vi "Práctica10_ProyectoFinal.vi"() -> ()   [LabVIEW 2021]
panel:
  out "Slide 3":u8(slide) scale=0.0..100.0
  out "Boolean 2":bool
  out "Slide 6":u8(slide) scale=0.0..100.0
  out "Boolean":bool
  out "Acorte 3":dbl(slide) scale=0.0..10.0
  out "Acorte 2":dbl(slide) scale=0.0..10.0
  out "Acorte":dbl(slide) scale=0.0..10.0
  out "Slide 5":u8(slide)
  out "Slide 5":u8(slide)
  out "Slide 5":u8(slide)
  in  "Tipo de papel":string(combo)
  out "Horno":dbl(knob) scale=0.0..100.0
  out "Lignina":dbl(slide) scale=0.0..500.0
  out "Lignina":bool
  out "Slide 5":u8(slide)
  out "Corte":bool
  out "Aplanado":bool
  out "Peroxido":dbl(slide) scale=0.0..500.0
  out "Slide 4":u8(slide)
  out "Slide 5":u8(slide)
  out "Blanquear":bool
  out "Limpieza":bool
  out "Slide 2":u8(slide) scale=0.0..4.0
  out "Distribución":bool
  out "Slide":u8(slide) scale=0.0..10.0 scale format="%_1g"
  out "Almacén":dbl(slide) scale=0.0..100.0
  out "Inicio":bool
  in  "Color Box":u32(colorbox)
  # "Tipo de papel"
  # "Almacén"
  # "Eliminado de lignina"
  # "Triturado"
  # "Aplanado"
  # "Blanqueado"
  # "Cortado"
  # "Distribuido"
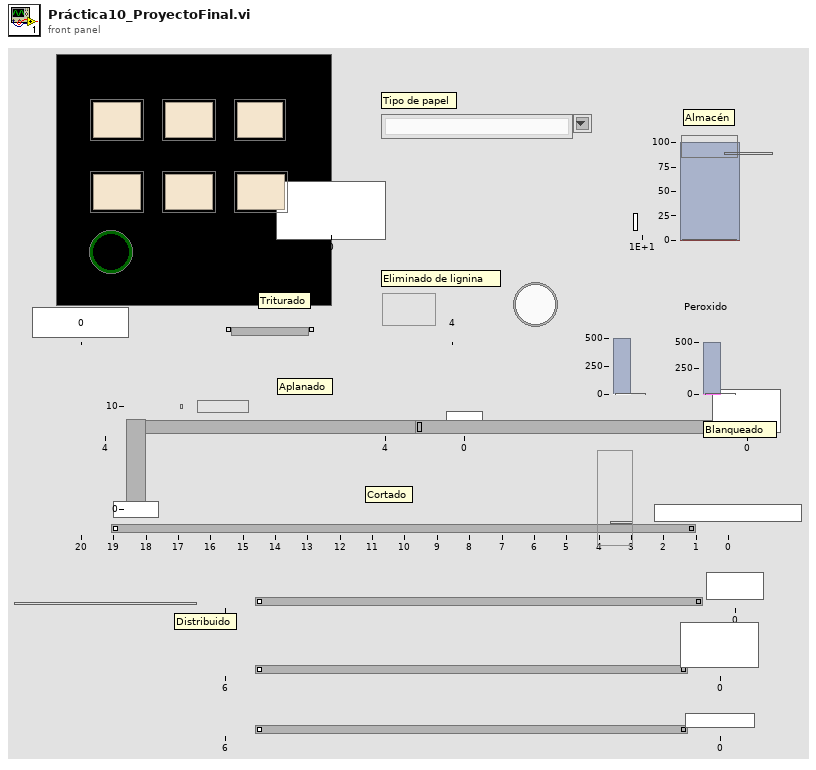
[diagram p1: front panel]
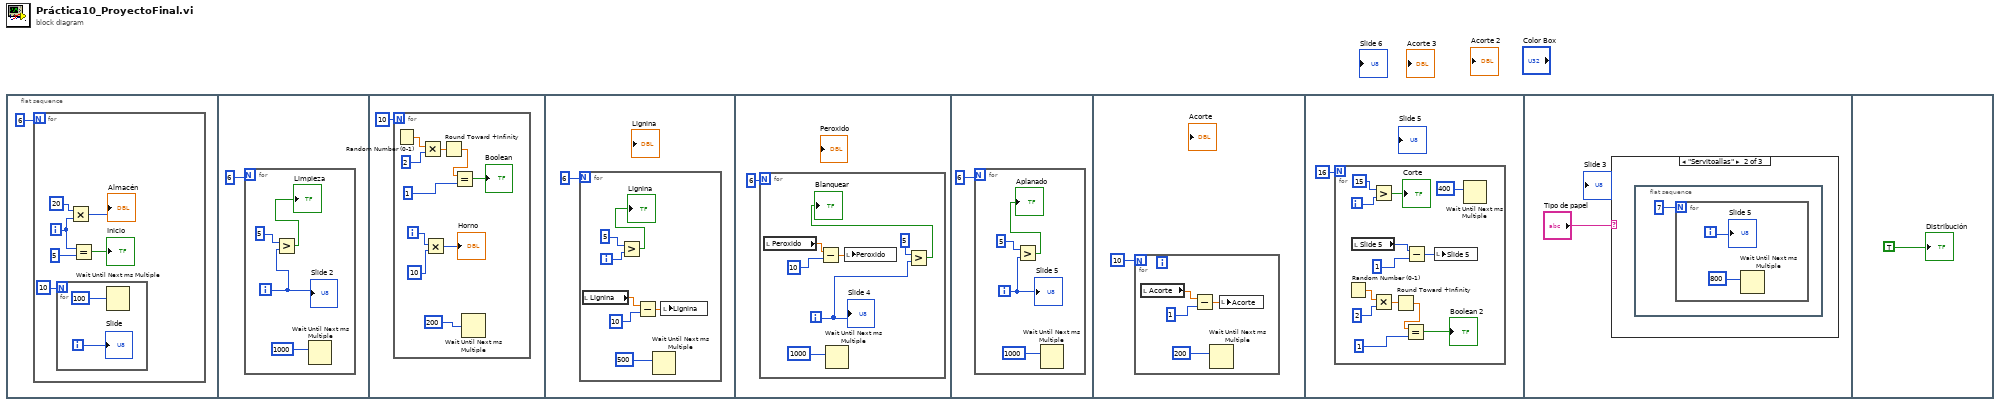
[diagram p0: block diagram]
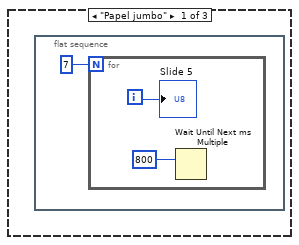
[diagram p2: hidden frame]
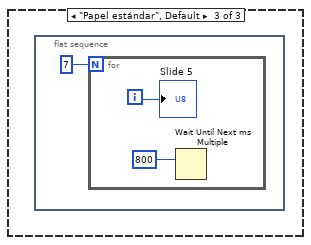
[diagram p3: hidden frame]
diagram:
  n1 = flat-sequence {
    frame #0 {
      n2 = for {
        N: 6 -> [_]
        i -> [w4]
        n3 = for {
          N: 10 -> [_]
          i -> [w8]
          n4 = Wait Until Next ms Multiple(millisecond multiple=100) -> ()  [unwired: 1 out]
          "Slide" <- w8
        }
        n5 = Multiply(x=20, y=w4) -> (x*y=→"Almacén":i32)
        n6 = Equal?(x=w4, y=5) -> (x = y?=→"Inicio":bool)
      }
    }
    frame #1 {
      n7 = for {
        N: 6 -> [_]
        i -> [w12]
        n8 = Greater?(x=5, y=w12) -> (0:→"Limpieza":bool)
        n9 = Wait Until Next ms Multiple(millisecond multiple=1000) -> ()  [unwired: 1 out]
        "Slide 2" <- w12
      }
    }
    frame #2 {
      n10 = for {
        N: 10 -> [_]
        i -> [w22]
        n11 = Random Number (0-1)() -> (number: 0 to 1=w21:dbl)
        n12 = Multiply(x=w21, y=2) -> (x*y=w17:dbl)
        n13 = Multiply(x=w22, y=10) -> (x*y=→"Horno":i32)
        n14 = Round Toward +Infinity(x=w17) -> (ceil(x): smallest int >= x=w16:dbl)
        n15 = Equal?(x=w16, y=1) -> (x = y?=→"Boolean":bool)
        n16 = Wait Until Next ms Multiple(millisecond multiple=200) -> ()  [unwired: 1 out]
      }
    }
    frame #3 {
      n17 = for {
        N: 6 -> [_]
        i -> [w30]
        n18 = local read "Lignina"() -> (w29:dbl)
        n19 = Greater?(x=5, y=w30) -> (0:→"Lignina":bool)
        n20 = Subtract(x=w29, y=10) -> (x-y=w27:dbl)
        n21 = Wait Until Next ms Multiple(millisecond multiple=500) -> ()  [unwired: 1 out]
        n22 = local write "Lignina"(w27) -> ()
      }
    }
    frame #4 {
      n23 = for {
        N: 6 -> [_]
        i -> [w35]
        n24 = local read "Peroxido"() -> (w41:dbl)
        n25 = Subtract(x=w41, y=10) -> (x-y=w39:dbl)
        n26 = Wait Until Next ms Multiple(millisecond multiple=1000) -> ()  [unwired: 1 out]
        n27 = local write "Peroxido"(w39) -> ()
        n28 = Greater?(x=5, y=w35) -> (0:→"Blanquear":bool)
        "Slide 4" <- w35
      }
    }
    frame #5 {
      n29 = for {
        N: 6 -> [_]
        i -> [w43]
        n30 = Greater?(x=5, y=w43) -> (0:→"Aplanado":bool)
        n31 = Wait Until Next ms Multiple(millisecond multiple=1000) -> ()  [unwired: 1 out]
        "Slide 5" <- w43
      }
    }
    frame #6 {
      n32 = for {
        N: 10 -> [_]
        n33 = local read "Acorte"() -> (w50:dbl)
        n34 = Subtract(x=w50, y=1) -> (x-y=w48:dbl)
        n35 = Wait Until Next ms Multiple(millisecond multiple=200) -> ()  [unwired: 1 out]
        n36 = local write "Acorte"(w48) -> ()
      }
    }
    frame #7 {
      n37 = for {
        N: 16 -> [_]
        i -> [w63]
        n38 = Random Number (0-1)() -> (number: 0 to 1=w58:dbl)
        n39 = local read "Slide 5"() -> (w61:u8)
        n40 = Greater?(x=15, y=w63) -> (0:→"Corte":bool)
        n41 = Multiply(x=w58, y=2) -> (x*y=w55:dbl)
        n42 = Round Toward +Infinity(x=w55) -> (ceil(x): smallest int >= x=w54:dbl)
        n43 = Equal?(x=w54, y=1) -> (x = y?=→"Boolean 2":bool)
        n44 = Subtract(x=w61, y=1) -> (x-y=w59:i32)
        n45 = local write "Slide 5"(w59) -> ()
        n46 = Wait Until Next ms Multiple(millisecond multiple=400) -> ()  [unwired: 1 out]
      }
    }
    frame #8 {
      n47 = case shown="\"Servitoallas\"" "Tipo de papel" {
        frame "Papel jumbo" {
          n48 = flat-sequence {
            frame #0 {
              n49 = for {
                N: 7 -> [_]
                i -> [w68]
                n50 = Wait Until Next ms Multiple(millisecond multiple=800) -> ()  [unwired: 1 out]
                "Slide 5" <- w68
              }
            }
          }
        }
        frame "Servitoallas" {
          n51 = flat-sequence {
            frame #0 {
              n52 = for {
                N: 7 -> [_]
                i -> [w71]
                n53 = Wait Until Next ms Multiple(millisecond multiple=800) -> ()  [unwired: 1 out]
                "Slide 5" <- w71
              }
            }
          }
        }
        frame "Papel estándar", Default {
          n54 = flat-sequence {
            frame #0 {
              n55 = for {
                N: 7 -> [_]
                i -> [w74]
                n56 = Wait Until Next ms Multiple(millisecond multiple=800) -> ()  [unwired: 1 out]
                "Slide 5" <- w74
              }
            }
          }
        }
      }
    }
    frame #9 {
      "Distribución" <- TRUE
    }
  }
